vi "verificarDatosImage.vi"(8 "error in":errorcluster, 11 "dataToWrite":T1) -> (0 "error out":errorcluster, 3 "dataToWriteModify":T2)   [LabVIEW 2014]
uses:
  <vilib>/addons/database/Auxilliary.llb/DB Tools Format Datetime String (Time Stamp).vi
  <vilib>/addons/database/NI_Database_API.lvlib
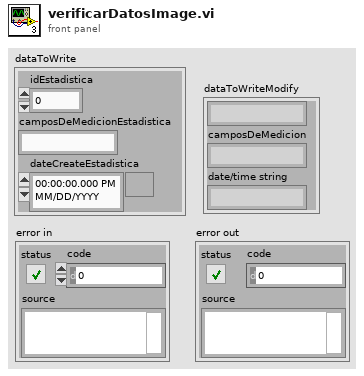
[diagram p1: front panel]
types:
  T1 = cluster{"idEstadistica":dbl, "camposDeMedicionEstadistica":string, "dateCreateEstadistica":timestamp}
  T2 = cluster{string, "camposDeMedicion":string, "date/time string":string}
  T3 = cluster{string, "camposDeMedicionEstadistica":string, "date/time string":string}
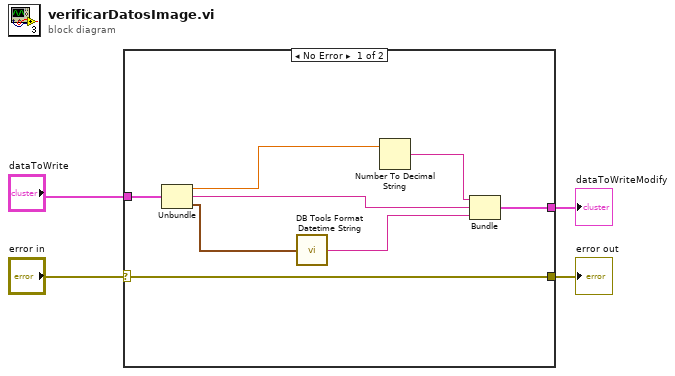
[diagram p0: block diagram]
diagram:
  n1 = case shown="No Error" "error in" {
    selector: "error in" -> [w5 w13]
    tunnel: "dataToWrite" -> [w12 _]
    tunnel: [w11 _] -> w3
    tunnel: [w5 w13] -> w1
    frame No Error {
      n2 = Unbundle(w12) -> ("idEstadistica"=w8:dbl, "camposDeMedicionEstadistica"=w7:string, "dateCreateEstadistica"=w6:timestamp)
      n3 = call-poly <vilib>:"DB Tools Format Datetime String.vi"("time stamp"=w6) -> ("date/time string"=w10:string)
      n4 = Number To Decimal String(number=w8) -> (decimal integer string=w9:string)  [unwired: 1 in]
      n5 = Bundle(w9, "camposDeMedicionEstadistica"=w7, "date/time string"=w10) -> (w11:T3)  [unwired: 1 in]
    }
    frame Error {
    }
  }
  "dataToWriteModify" <- w3
  "error out" <- w1
